vi "Send Configure Reference Levels [WM].vi"(6 "high reference (90.0%)":dbl=90.0 format="%.3f", 7 "Message Priority (Normal)":T1=enum."Normal", 8 "error in (no error)":errorcluster, 9 "mid reference (50.0%)":dbl=50.0 format="%.3f", 10 "low reference (10.0%)":dbl=10.0 format="%.3f", 11 "Message Enqueuer":refnum<class "Message Enqueuer.lvclass">) -> (0 "error out":errorcluster, 3 "Message Enqueuer out":refnum<class "Message Enqueuer.lvclass">)   [LabVIEW 2015, in "CS++Scope.lvlib" / "Configure Reference Levels [WM] Msg.lvclass"]
doc: "Sends the <B>CS++Scope.lvlib:Configure Reference Levels [WM] Msg.lvclass</B> message.\n\n<B>CS++Scope.lvlib:CS++Scope.lvclass:Configure Reference Levels [WM].vi</B> Description:\n\nThis VI configures the reference levels for waveform measurements. \n\nYou must call this VI before you call the IviScope Read Waveform Measurement [WM] or IviScope Fetch Waveform Measurement [WM] to take a rise time, fall time, width negative, width positive, duty cycle negative, duty cycle positive, preshoot, or overshoot measurement.\n\nNotes:\n\n(1) This VI is part of the IviScopeWaveformMeasurement [WM] extension group."
uses:
  Configure Reference Levels [WM] Msg.lvclass
  <vilib>/ActorFramework/Message Enqueuer/Message Enqueuer.lvclass
  <vilib>/ActorFramework/Message Enqueuer/Message Priority.ctl
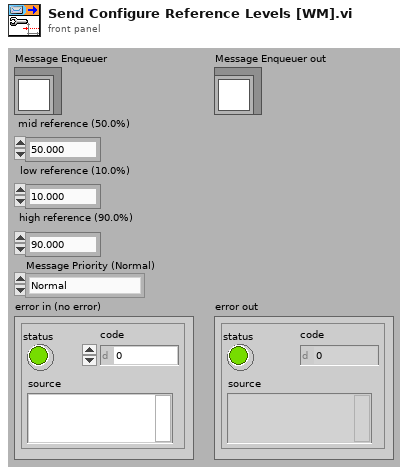
[diagram p1: front panel]
types:
  T1 = typedef "Actor Framework.lvlib/Message Enqueuer.lvclass/Message Priority.ctl" = enum16{"Low", "Normal", "High"}
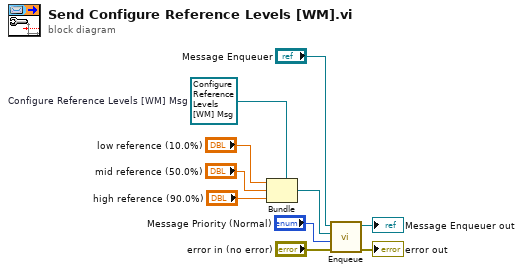
[diagram p0: block diagram]
diagram:
  w4 = refnum<class "Configure Reference Levels [WM] Msg.lvclass"> refnum  # Configure Reference Levels [WM] Msg
  n1 = Bundle(cluster=w4, "low reference (10.0%)", "mid reference (50.0%)", "high reference (90.0%)") -> (w7:refnum<class "Configure Reference Levels [WM] Msg.lvclass">)
  n2 = call <vilib>:"Enqueue.vi"("error in (no error)"="error in (no error)", "Message Priority (Normal)"="Message Priority (Normal)", "Message"=w7, "Message Enqueuer in"="Message Enqueuer") -> ("error out"=→"error out":errorcluster, "Message Enqueuer out"=→"Message Enqueuer out":refnum<class "Message Enqueuer.lvclass">)  [unwired: 6 in]
